vi "Get Sensor Data.vi"(8 "error in":errorcluster, 9 "sensor_id":i32, 10 "test_num":i32, 11 "conn":u32) -> (0 "error out":errorcluster, 1 "number":dbl, 2 "field_value":string, 3 "PQresultStatus":T1(ring))   [LabVIEW 2017]
uses:
  PostgreSQL2LabVIEW/libpqlv/libpqlv.lvlib
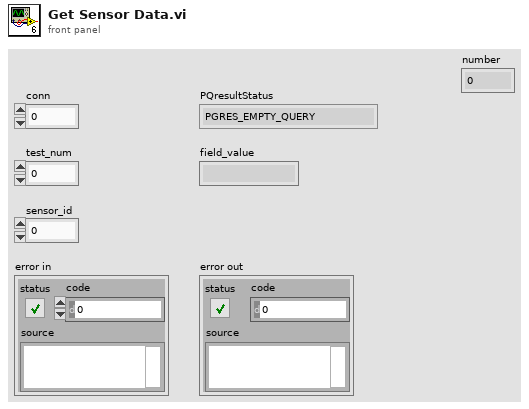
[diagram p1: front panel]
types:
  T1 = enum16{"PGRES_EMPTY_QUERY", "PGRES_COMMAND_OK", "PGRES_TUPLES_OK", "PGRES_COPY_OUT", "PGRES_COPY_IN", "PGRES_BAD_RESPONSE", "PGRES_NONFATAL_ERROR", "PGRES_FATAL_ERROR"}
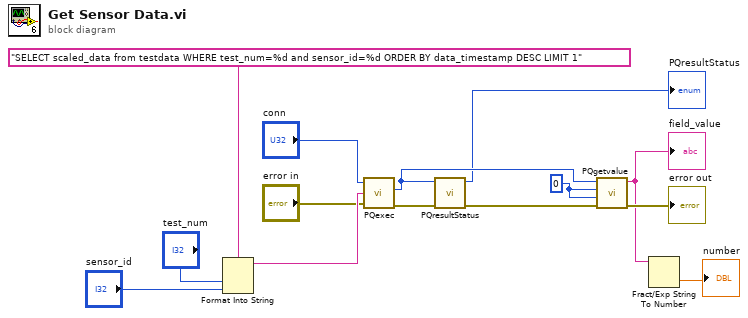
[diagram p0: block diagram]
diagram:
  w1 = 0 ("row_number")
  n1 = Format Into String(format string="SELECT scaled_data from testdata WHERE test_num=%d and sensor_id=%d ORDER BY data_timestamp DESC LIMIT 1", "test_num", "sensor_id") -> (resulting string=w13:string)  [unwired: 2 in, 1 out]
  n2 = call "PQexec.vi"("conn"="conn", "query"=w13, "error in (no error)"="error in") -> ("PGresult"=w11:u32, "error out"=w10:errorcluster)  [unwired: 2 in]
  n3 = call "PQresultStatus.vi"("error in (no error)"=w10, "res"=w11) -> ("error out"=w7:errorcluster, "PQresultStatus"=→"PQresultStatus":T1)  [unwired: 8 in]
  n4 = call "PQgetvalue.vi"("error in (no error)"=w7, "column_number"=w1, "row_number"=w1, "res"=w11) -> ("error out"=→"error out":errorcluster, "field_value"=w3:string)  [unwired: 6 in]
  "field_value" <- w3
  n5 = Fract/Exp String To Number(string=w3) -> (number=→"number":dbl)  [unwired: 3 in, 1 out]
